vi "SDG60ConfPRBS.vi"(2 "Differental mode (0: Off)":u16(ring) items=["Off", "On"], 4 "Offset (0.00 V)":dbl min=-10.0 max=10.0 format="%#_15g", 5 "BitRate/Period (T:BitRate)":bool=TRUE, 6 "Amplitude (1 Vpp)":dbl=1.0, 7 "Length (3)":u16=3, 8 "error in (no error)":errorcluster, 9 "Bit Rate/Period (1000 bits/second)":dbl=1000.0 format="%#_15g", 10 "Channel (1: Ch1)":u16(ring)=1 items=["Channel 1"=1, "Channel 2"=2], 11 "VISA resource name":refnum<visa-resource-name>="USB0::0xF4EC::0x1101::SDG6XEBC5R0119::INSTR") -> (0 "error out":errorcluster, 3 "VISA resource name out":refnum<visa-resource-name>)   [LabVIEW 2018]
doc: "Configures PRBS waveform and parameters.\n\nNote:\nThis VI only supports SDG6000X series."
panel:
  in  "Edge Time (10 ns)":dbl=1e-08 format="%#_16g"
  # "Logic Level changable only via front panel"
  # "Range 1 mbit/sec to 300 Mbits/sec\n10 digits precision"
  # "Range: 3-32\nActual PRBS length = 2^(LENGTH)-1"
  # "Range:1ns - 1ms Max depends on period\n6 digits precision"
  # "Range: 2mVpp-20Vpp\n6 digits precision"
  # "Range +/- 9.999V\n6 digits precision"
  # "Will be really differential when both ch\noutputs are ON. Switching outputs OFF ruins phase relation of the channels"
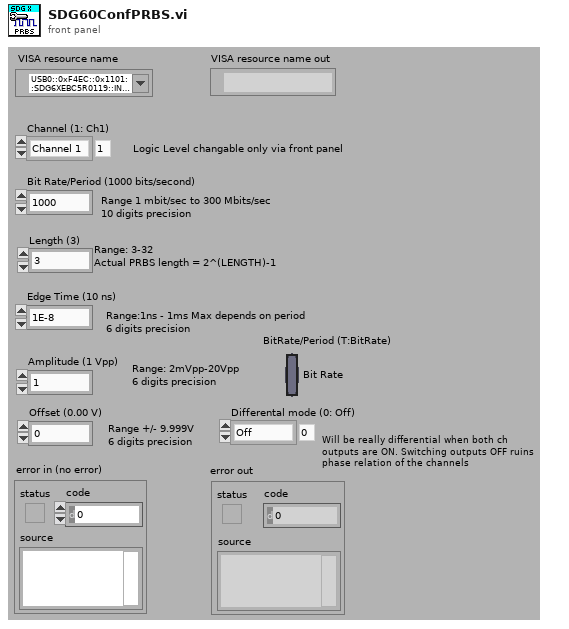
[diagram p1: front panel]
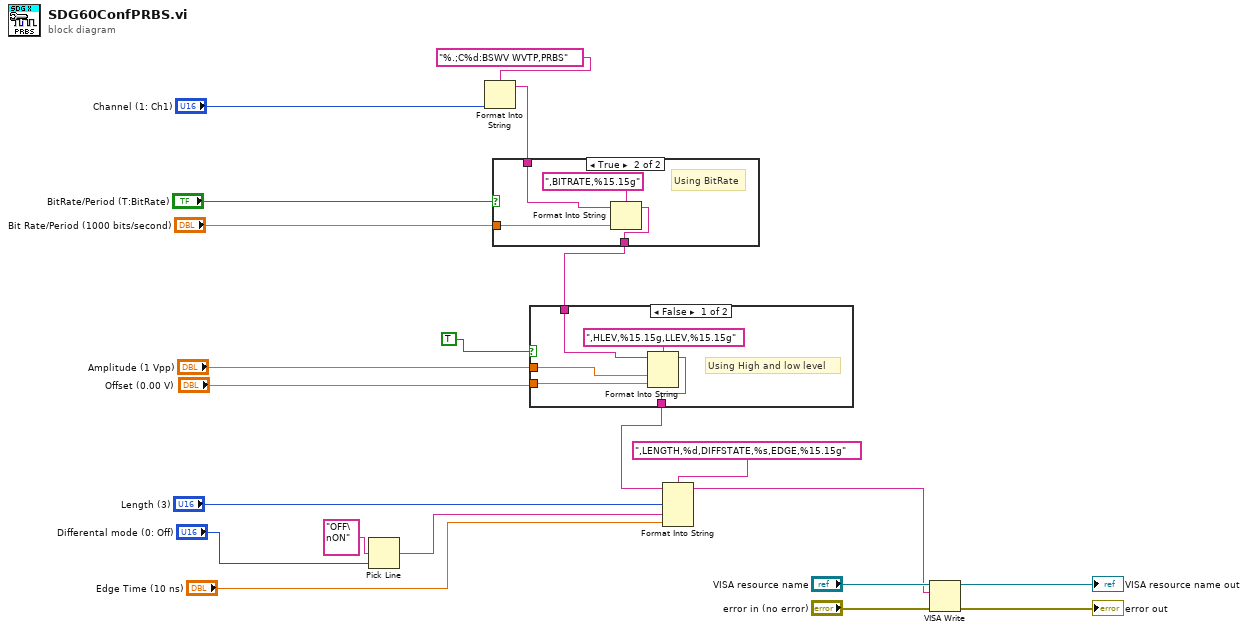
[diagram p0: block diagram]
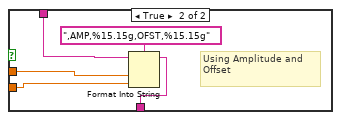
[diagram p2: hidden frame]
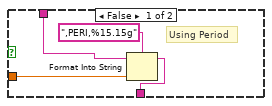
[diagram p3: hidden frame]
diagram:
  n1 = Pick Line(multi-line string="OFF\nON", line index="Differental mode (0: Off)") -> (output string=w3:string)  [unwired: 1 in]
  n2 = Format Into String(format string="%.;C%d:BSWV WVTP,PRBS", "Channel (1: Ch1)") -> (resulting string=w6:string)  [unwired: 2 in, 1 out]
  n3 = case shown="True" "BitRate/Period (T:BitRate)" {
    tunnel: w6 -> [w23 w27]
    tunnel: [w22 w26] -> w15
    tunnel: "Bit Rate/Period (1000 bits/second)" -> [w24 w28]
    frame False {
      # "Using Period"
      n4 = Format Into String(format string=",PERI,%15.15g", initial string=w23, w24) -> (resulting string=w22:string)  [unwired: 1 in, 1 out]
    }
    frame True {
      # "Using BitRate"
      n5 = Format Into String(format string=",BITRATE,%15.15g", initial string=w27, w28) -> (resulting string=w26:string)  [unwired: 1 in, 1 out]
    }
  }
  n6 = case shown="False" TRUE {
    tunnel: w15 -> [w32 w37]
    tunnel: [w31 w36] -> w9
    tunnel: "Amplitude (1 Vpp)" -> [w33 w38]
    tunnel: "Offset (0.00 V)" -> [w30 w35]
    frame False {
      # "Using High and low level"
      n7 = Format Into String(format string=",HLEV,%15.15g,LLEV,%15.15g", initial string=w32, w33, w30) -> (resulting string=w31:string)  [unwired: 1 in, 1 out]
    }
    frame True {
      # "Using Amplitude and Offset"
      n8 = Format Into String(format string=",AMP,%15.15g,OFST,%15.15g", initial string=w37, w38, w35) -> (resulting string=w36:string)  [unwired: 1 in, 1 out]
    }
  }
  n9 = Format Into String(format string=",LENGTH,%d,DIFFSTATE,%s,EDGE,%15.15g", initial string=w9, "Length (3)", w3, "Edge Time (10 ns)") -> (resulting string=w1:string)  [unwired: 1 in, 1 out]
  n10 = VISA Write(VISA resource name="VISA resource name", write buffer=w1, error in (no error)="error in (no error)") -> (VISA resource name out=→"VISA resource name out":refnum<visa-resource-name>, error out=→"error out":errorcluster)  [unwired: 1 out]
